vi "12.1 Determine Warning (SubVI).vi"(8 "Error In":errorcluster, 11 "Weather Data In":T1) -> (0 "Error Out":errorcluster, 3 "Weather Data Out":T1)   [LabVIEW 2019]
uses:
  13.1 Weather Data.ctl
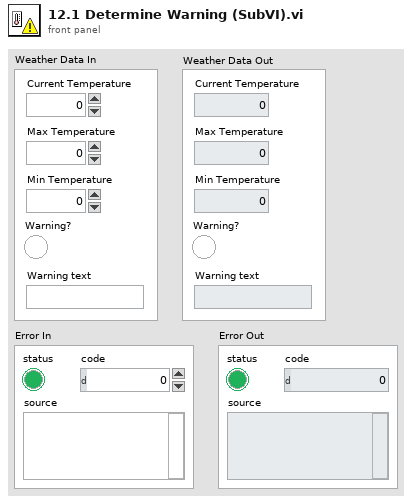
[diagram p1: front panel]
types:
  T1 = typedef "13.1 Weather Data.ctl" = cluster{"Current Temperature":dbl, "Max Temperature":dbl, "Min Temperature":dbl, "Warning?":bool, "Warning text":string}
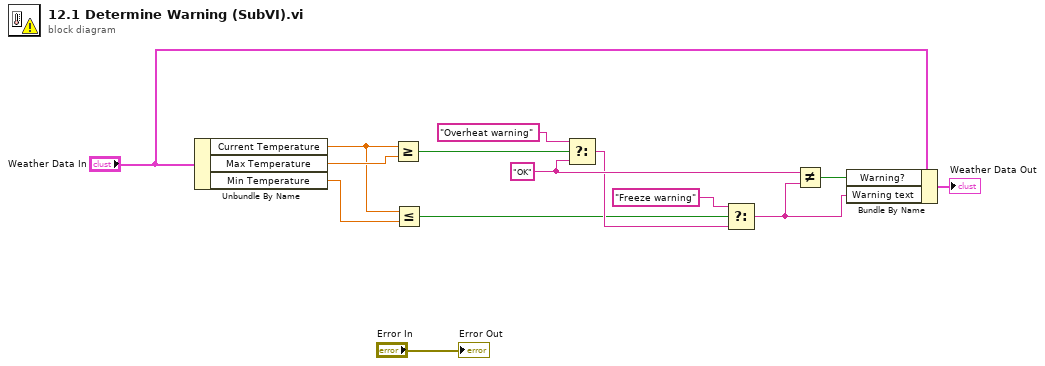
[diagram p0: block diagram]
diagram:
  w14 = "OK"
  n1 = Unbundle By Name("Weather Data In") -> ("Current Temperature"=w5:dbl, "Max Temperature"=w7:dbl, "Min Temperature"=w6:dbl)
  n2 = Greater Or Equal?(x=w5, y=w7) -> (x >= y?=w9:bool)
  n3 = Less Or Equal?(x=w5, y=w6) -> (x <= y?=w11:bool)
  n4 = Select(t="Overheat warning", s=w9, f=w14) -> (s? t:f=w13:string)
  n5 = Select(t="Freeze warning", s=w11, f=w13) -> (s? t:f=w2:string)
  n6 = Not Equal?(x=w14, y=w2) -> (x != y?=w3:bool)
  n7 = Bundle By Name(cluster="Weather Data In", "Warning?"=w3, "Warning text"=w2) -> (→"Weather Data Out":T1)
  "Error Out" <- "Error In"
